vi "CalcDistanceFromEnd.vi"(11 "Path":cluster{"x":dbl, "y":dbl}[](array[cluster])=[{"x"=0.0, "y"=0.0}, {"x"=270.0, "y"=0.0}, {"x"=290.0, "y"=-50.0}]) -> (3 "DistancesToEnd":dbl[](array[numeric]))   [LabVIEW 2017]
doc: "Returns an array describing how far each point is away from the end of the path, along the path (not straight line distance)"
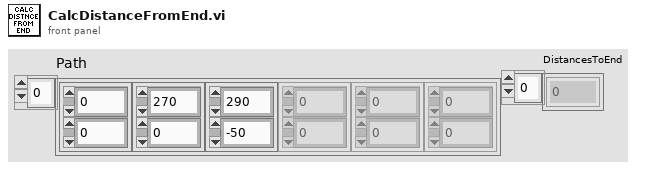
[diagram p1: front panel]
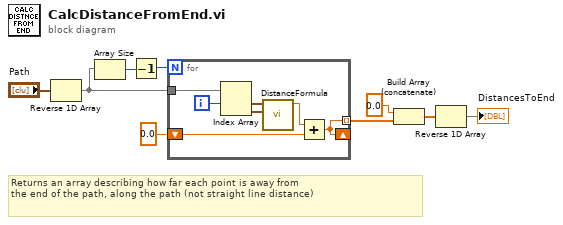
[diagram p0: block diagram]
diagram:
  # "Returns an array describing how far each point is away from\nthe end of the path, along the path (not straight line distance)"
  n1 = Reverse 1D Array(array="Path") -> (reversed array=w7:cluster{"x":dbl, "y":dbl}[])
  n2 = Array Size(array=w7) -> (size(s)=w6:i32)
  n3 = Decrement(x=w6) -> (x-1=w5:i32)
  n4 = for {
    N: w5 -> [_]
    tunnel: w7 -> [w16]
    shift-right: [w10] -> _
    shift-left: 0.0 -> [w11]
    tunnel: [w10] -> w3 mode=indexing
    i -> [w15]
    n5 = Index Array(array=w16, index #1=w15) -> (element #1=w14:cluster{"x":dbl, "y":dbl}, element #2=w13:cluster{"x":dbl, "y":dbl})  [unwired: 1 in]
    n6 = call "DistanceFormula.vi"("Point 2"=w13, "Point 1"=w14) -> ("Distance"=w12:dbl)  [unwired: 9 in]
    n7 = Add(x=w12, y=w11) -> (x+y=w10:dbl)
  }
  n8 = Build Array (concatenate)(0.0 ("element"), w3) -> (w2:dbl[])
  n9 = Reverse 1D Array(array=w2) -> (reversed array=→"DistancesToEnd":dbl[])
